vi "Pololu-Set Acceleration.vi"(4 "User Units Max":u16, 5 "Servo Units Max":u16, 6 "User Units Min":u16, 7 "Servo Units Min":u16, 8 "error in":errorcluster, 9 "Servo Chan":u16, 10 "Acceleration (deg/sec^2)":u16, 11 "VISA resource name":refnum<visa-resource-name>) -> (0 "error out":errorcluster)   [LabVIEW 2018]
uses:
  <vilib>/Instr/_visa.llb/VISA Configure Serial Port (Instr).vi
panel:
  out "sent string":string
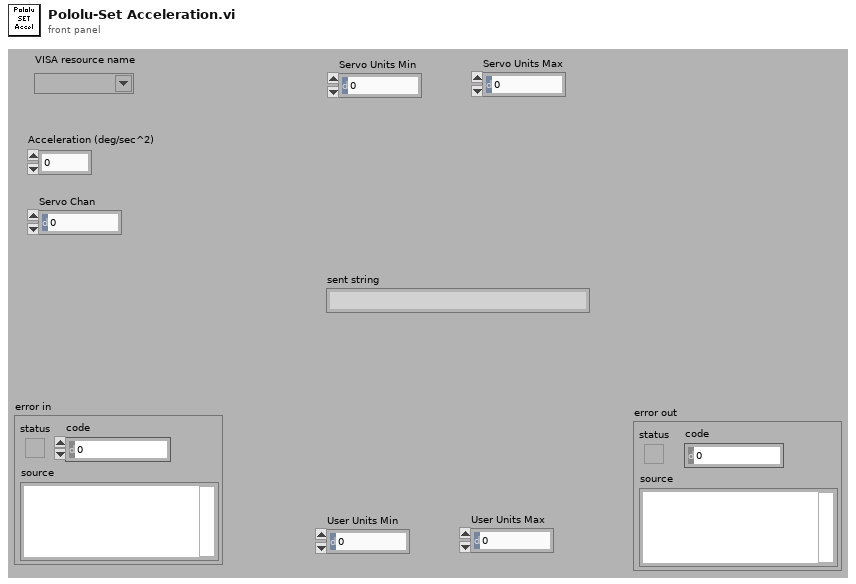
[diagram p1: front panel]
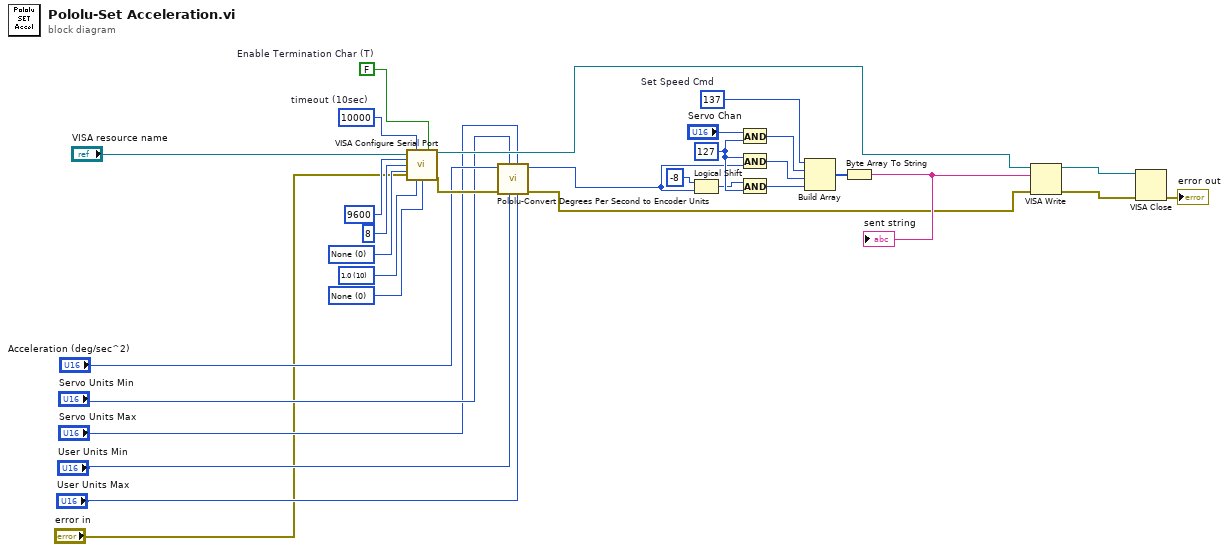
[diagram p0: block diagram]
diagram:
  w7 = u16 0 items=["None"=0, "XON/XOFF"=1, "RTS/CTS"=2, "DTR/DSR"=4] ("flow control")
  w8 = u16 10 items=["1.0"=10, "1.5"=15, "2.0"=20] ("stop bits")
  w9 = u16 0 items=["None", "Odd", "Even", "Mark", "Space"] ("parity")
  w12 = FALSE  # Enable Termination Char (T)
  w13 = u32 10000  # timeout (10sec)
  w22 = u8 137  # Set Speed Cmd
  w24 = u8 127
  n1 = call-poly "VISA Configure Serial Port"("VISA resource name"="VISA resource name", "timeout (10sec)"=w13, "Enable Termination\nChar (T)"=w12, "baud rate (9600)"=u32 9600 ("baud rate"), "data bits (8)"=u16 8 ("data bits"), "parity (0:none)"=w9, "error in (no error)"="error in", "stop bits (10: 1 bit)"=w8, "flow control (0:none)"=w7) -> ("VISA resource name out"=w28:refnum<visa-resource-name>, "error out"=w16:errorcluster)  [unwired: 5 out]
  n2 = call "Pololu-Convert Degrees Per Second to Encoder Units.vi"("Degree Max"="User Units Max", "Encoder Units Max"="Servo Units Max", "Degree Min"="User Units Min", "Encoder Units Min"="Servo Units Min", "Error In"=w16, "Speed (deg/sec)"="Acceleration (deg/sec^2)") -> ("Error Out"=w15:errorcluster, "Speed Encoder Units"=w17:u16)  [unwired: 4 in]
  n3 = Logical Shift(y=i8 -8, x=w17) -> (x << y=w21:u16)
  n4 = And(x="Servo Chan", y=w24) -> (x .and. y?=w25:u16)
  n5 = And(x=w24, y=w17) -> (x .and. y?=w26:u16)
  n6 = And(x=w21, y=w24) -> (x .and. y?=w27:u16)
  n7 = Build Array(w22, w25, w26, w27) -> (w18:u16[])
  n8 = Byte Array To String(unsigned byte array=w18) -> (string=w19:string)
  "sent string" <- w19
  n9 = VISA Write(VISA resource name=w28, write buffer=w19, error in (no error)=w15) -> (VISA resource name out=w31:refnum<visa-resource-name>, error out=w30:errorcluster)  [unwired: 1 out]
  n10 = VISA Close(VISA resource name=w31, error in (no error)=w30) -> (error out=→"error out":errorcluster)
